vi "Create Instrument Addon.vi"(8 "error in (no error)":errorcluster, 9 "PCL decimation":u16=1, 10 "protocol in":refnum<class "Protocol Parent.lvclass">, 11 "target in":refnum<k24>) -> (0 "error out":errorcluster, 2 "instrument addon refnum":T1=18446744073709551615 format="%.0x", 3 "target out":refnum<k24>)   [LabVIEW 2018, in "Instrument Addon Scripting API.lvlib"]
doc: "Creates an Instrument Addon Custom Device using the specified settings."
uses:
  Instrument Addon Scripting API.lvlib
  NationalInstruments.VeriStand.SystemDefinitionAPI
  Addon/Support Libraries/Protocols.lvlibp/Protocol Parent/Protocol Parent.lvclass
  <vilib>/NI Veristand/Custom Device API/Custom Device Item Ref.ctl
  <vilib>/NI Veristand/Custom Device API/Custom Device API.lvlib
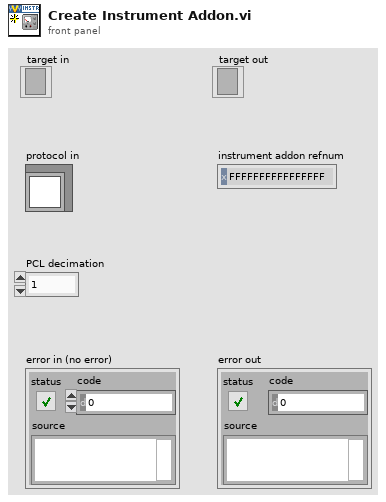
[diagram p1: front panel]
types:
  T1 = typedef "Custom Device API.lvlib/Custom Device Item Ref.ctl" = u64
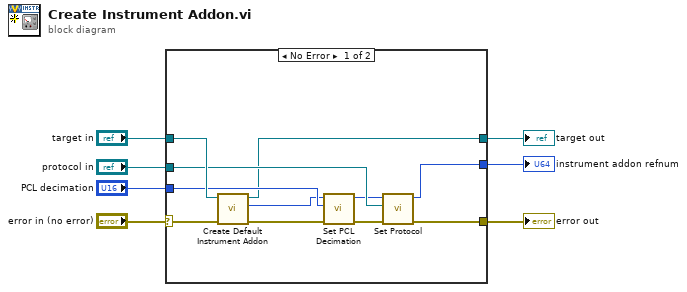
[diagram p0: block diagram]
diagram:
  n1 = case shown="No Error" "error in (no error)" {
    selector: "error in (no error)" -> [w17 w19]
    tunnel: "target in" -> [w18 w20]
    tunnel: "PCL decimation" -> [w15 _]
    tunnel: "protocol in" -> [w12 _]
    tunnel: [w10 w20] -> w3
    tunnel: [w9 w19] -> w1
    tunnel: [w8 _] -> w2
    frame No Error {
      n2 = call "Create Default Instrument Addon.vi"("Error In"=w17, "Target In"=w18) -> ("Error Out"=w16:errorcluster, "Instrument Addon Refnum"=w13:T1, "Target Out"=w10:refnum<k24>)  [unwired: 7 in]
      n3 = call "Set PCL Decimation.vi"("error in (no error)"=w16, "PCL decimation"=w15, "instrument addon refnum in"=w13) -> ("error out"=w14:errorcluster, "instrument addon refnum"=w11:T1)  [unwired: 7 in]
      n4 = call "Set Protocol.vi"("error in (no error)"=w14, "protocol"=w12, "instrument addon refnum in"=w11) -> ("error out"=w9:errorcluster, "instrument addon refnum out"=w8:T1)  [unwired: 7 in]
    }
    frame Error {
    }
  }
  "target out" <- w3
  "instrument addon refnum" <- w2
  "error out" <- w1
